vi "OC2 Read Setpoint.vi"(7 "enable":bool, 8 "error in (no error)":errorcluster, 9 "Read  setpoint values":T1 {"C coeff deg" format="%.2f"; "Rate deg/V" format="%.3f"; "X coeff deg/V" format="%.2f"; "pot offset" format="%.2f"; "value" format="%.3f"; "pot range" format="%.2f"; "Setpoint" items=["Pot", "Value"]}, 11 "VISA resource name":refnum<visa-resource-name>) -> (0 "error out":errorcluster, 1 "Read  setpoint values out":T1 {"C coeff deg" format="%.2f"; "Rate deg/V" format="%.3f"; "X coeff deg/V" format="%.2f"; "pot offset" format="%.2f"; "value" format="%.3f"; "pot range" format="%.2f"; "Setpoint" items=["Pot", "Value"]}, 3 "dup VISA resource name":refnum<visa-resource-name>)   [LabVIEW 2009]
panel:
  in  "Command":string
  out "write data":string
  # "Set setpoint variables"
  # "V1.02"
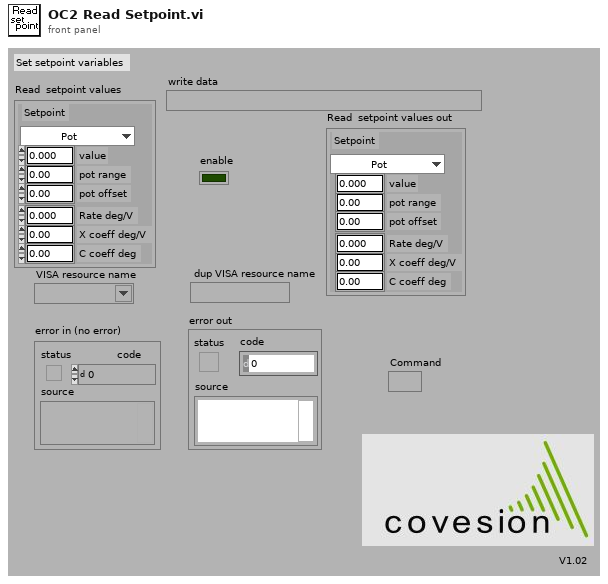
[diagram p1: front panel]
types:
  T1 = cluster{"Setpoint":u16, "pot range":dbl, "value":dbl, "pot offset":dbl, "X coeff deg/V":dbl, "Rate deg/V":dbl, "C coeff deg":dbl}
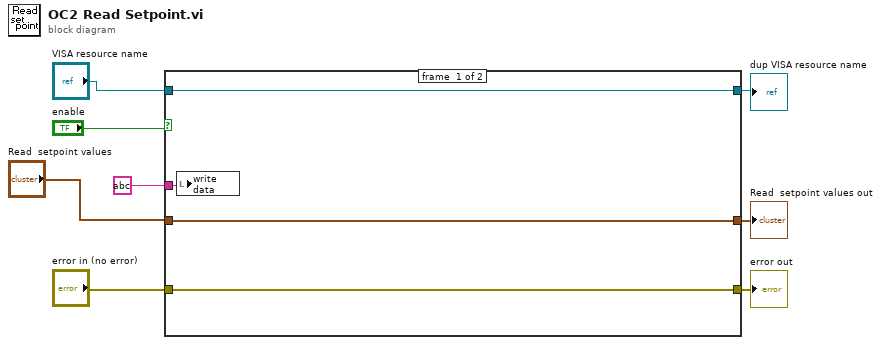
[diagram p0: block diagram]
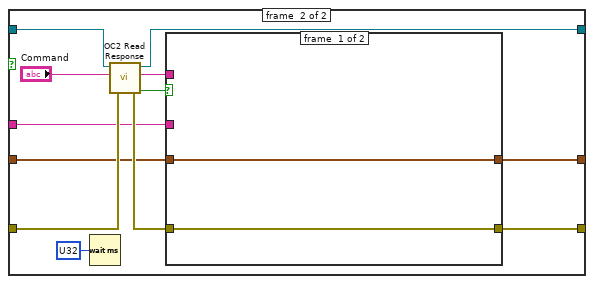
[diagram p2: hidden frame]
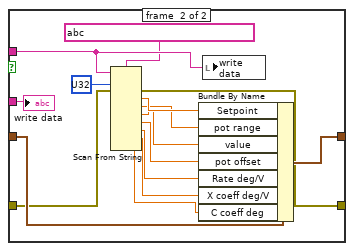
[diagram p3: hidden frame]
diagram:
  n1 = case shown="True" "enable" {
    tunnel: "VISA resource name" -> [w12 w23]
    tunnel: [w12 w21] -> w4
    tunnel: "error in (no error)" -> [w11 w19]
    tunnel: [w11 w18] -> w6
    tunnel: [w10 w17] -> w2
    tunnel: "Read  setpoint values" -> [w10 w16]
    tunnel: string ? ("Rx string") -> [w9 w15]
    frame #0 {
      n2 = local write "write data"(w9) -> ()
    }
    frame #1 {
      n3 = Wait (ms)(milliseconds to wait=u32 ?) -> ()  [unwired: 1 out]
      n4 = call "OC2 Read Response.vi"("error in (no error)"=w19, "Command"="Command", "VISA resource name"=w23) -> ("RX packet ok"=w22:bool, "error out"=w20:errorcluster, "output string"=w24:string, "dup VISA resource name"=w21:refnum<visa-resource-name>)  [unwired: 1 in]
      n5 = case shown="True" w22 {
        tunnel: w24 -> [_ w38]
        tunnel: w20 -> [w26 w29]
        tunnel: [w26 w27] -> w18
        tunnel: [w25 w28] -> w17
        tunnel: w16 -> [w25 w41]
        tunnel: w15 -> [_ w39]
        frame #0 {
        }
        frame #1 {
          n6 = Scan From String(format string=string ?, input string=w38, initial scan location=u32 ?, error in=w29) -> (error out=w27:errorcluster, output 1=w36:dbl, output 2=w35:dbl, output 3=w34:dbl, output 4=w33:dbl, output 5=w32:dbl, output 6=w31:dbl, output 7=w30:dbl)  [unwired: 7 in, 2 out]
          n7 = Bundle By Name(cluster=w41, "Setpoint"=w36, "pot range"=w35, "value"=w34, "pot offset"=w33, "Rate deg/V"=w32, "X coeff deg/V"=w31, "C coeff deg"=w30) -> (w28:T1)
          n8 = local write "write data"(w38) -> ()
          "write data" <- w39
        }
      }
    }
  }
  "dup VISA resource name" <- w4
  "error out" <- w6
  "Read  setpoint values out" <- w2
